vi "KlingerV2 DecodeStatus.vi"(0 "Axe":u8(ring) items=["W", "X", "Y", "Z"], 2 "Message Cont":string caption="Message de statut", 3 "error in":errorcluster) -> (4 "PLimit":bool caption="Limite +", 5 "Moving":bool caption="Déplacement\nen cours", 6 "Position":dbl format="%#.1f", 7 "Statut":bool, 8 "NLimit":bool caption="Limite -", 10 "error out":errorcluster)   [LabVIEW 2012]
doc: "Ce VI décode le message de statut du contrôleur et rapporte les informations pour l'axe désiré"
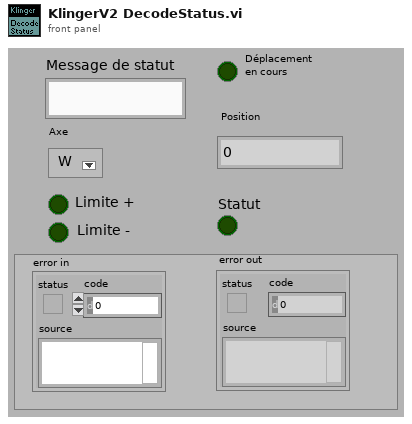
[diagram p1: front panel]
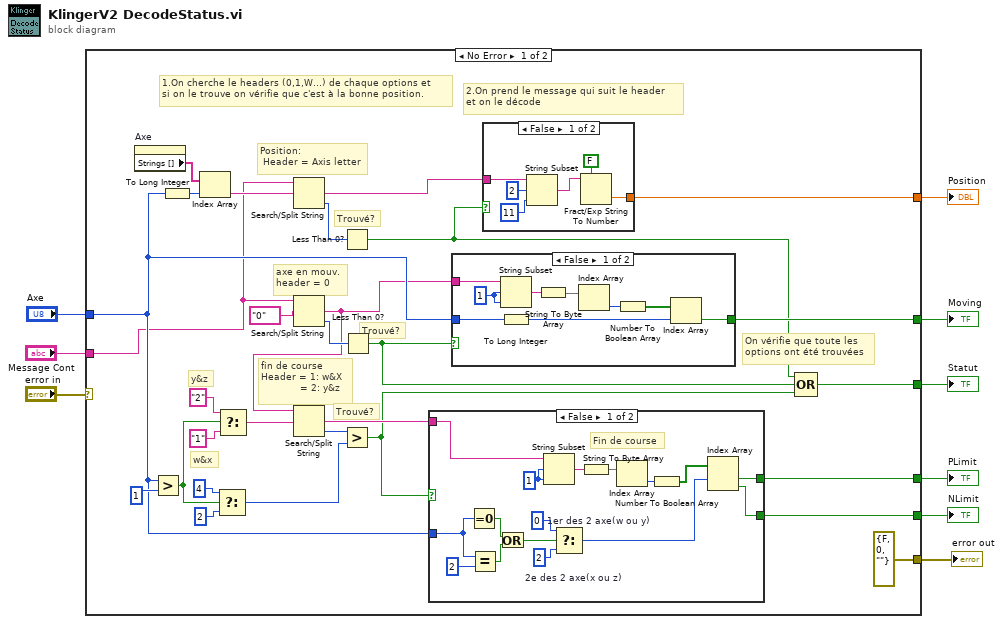
[diagram p0: block diagram]
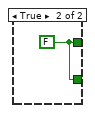
[diagram p2: hidden frame]
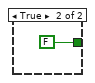
[diagram p3: hidden frame]
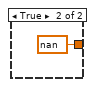
[diagram p4: hidden frame]
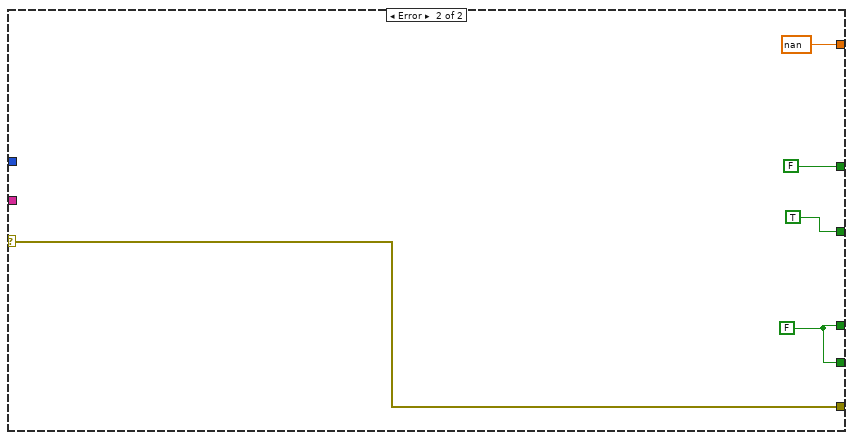
[diagram p5: hidden frame]
diagram:
  n1 = case shown="No Error" "error in" {
    selector: "error in" -> [_ w75]
    tunnel: [w35 nan] -> w9
    tunnel: [w34 FALSE] -> w8
    tunnel: "Axe" -> [w16 _]
    tunnel: [errorcluster {"status"=FALSE, "code"=0, "source"=""} ("error IO") w75] -> w6
    tunnel: [w17 TRUE ("Statut")] -> w5
    tunnel: "Message Cont" -> [w11 _]
    tunnel: [w19 w73] -> w2
    tunnel: [w18 w73] -> w1
    frame No Error {
      # "2.On prend le message qui suit le header \net on le décode"
      # "1.On cherche le headers (0,1,W...) de chaque options et\nsi on le trouve on vérifie que c'est à la bonne position."
      # "Trouvé?"
      # "Trouvé?"
      # "Trouvé?"
      # "On vérifie que toute les \noptions ont été trouvées"
      # "w&x"
      # "y&z"
      # "fin de course\nHeader = 1: w&X\n             = 2: y&z"
      # "Position:\n Header = Axis letter"
      # "axe en mouv.\nheader = 0"
      n2 = property on="Axe" class="Ring (strict)"() -> ("Strings []"=w33:string[])  [unwired: 2 in, 2 out]
      n3 = Greater?(x=w16, y=u8 1) -> (0:w23:bool)
      n4 = To Long Integer(number=w16) -> (32bit integer=w38:i32)
      n5 = Index Array(array=w33, index=w38) -> (element=w37:string)
      n6 = Select(t=4 ("y"), s=w23, f=2 ("y")) -> (s? t:f=w21:i32)
      n7 = Select(t="2" ("search string/char (-)"), s=w23, f="1" ("search string/char (-)")) -> (s? t:f=w22:string)
      n8 = Search/Split String(string=w11, search string/char (-)=w37) -> (match + rest of string=w36:string, offset of match=w32:i32)  [unwired: 1 in, 1 out]
      n9 = Search/Split String(string=w11, search string/char (-)="0") -> (match + rest of string=w10:string, offset of match=w30:i32)  [unwired: 1 in, 1 out]
      n10 = Search/Split String(string=w10, search string/char (-)=w22) -> (match + rest of string=w20:string, offset of match=w29:i32)  [unwired: 1 in, 1 out]
      n11 = Less Than 0?(x=w32) -> (x < 0?=w14:bool)
      n12 = Greater?(x=w29, y=w21) -> (0:w12:bool)
      n13 = Less Than 0?(x=w30) -> (x < 0?=w13:bool)
      n14 = case shown="False" w12 {
        tunnel: w20 -> [w43 _]
        tunnel: [w41 w55] -> w19
        tunnel: [w40 w55] -> w18
        tunnel: w16 -> [w39 _]
        frame False {
          w52 = 2  # 2e des 2 axe(x ou z)
          w53 = 0  # 1er des 2 axe(w ou y)
          w44 = 1 ("offset (0)")
          # "Fin de course"
          n15 = Equal To 0?(x=w39) -> (x = 0?=w51:bool)
          n16 = Equal?(x=w39, y=u8 2) -> (x = y?=w50:bool)
          n17 = Or(x=w51, y=w50) -> (x .or. y?=w48:bool)
          n18 = String Subset(string=w43, offset (0)=w44, length (rest)=w44) -> (substring=w47:string)
          n19 = Select(t=w53, s=w48, f=w52) -> (s? t:f=w42:i32)
          n20 = String To Byte Array(string=w47) -> (unsigned byte array=w46:u8[])
          n21 = Index Array(array=w46) -> (element=w45:u8)  [unwired: 1 in]
          n22 = Number To Boolean Array(number=w45) -> (Boolean array=w54:bool[])
          n23 = Index Array(array=w54, index #1=w42) -> (element #1=w41:bool, element #2=w40:bool)  [unwired: 1 in]
        }
        frame True {
          w55 = FALSE
        }
      }
      n24 = case shown="False" w13 {
        tunnel: [w61 FALSE] -> w34
        tunnel: w10 -> [w59 _]
        tunnel: w16 -> [w56 _]
        frame False {
          w58 = 1 ("offset (0)")
          n25 = String Subset(string=w59, offset (0)=w58, length (rest)=w58) -> (substring=w60:string)
          n26 = To Long Integer(number=w56) -> (32bit integer=w57:i32)
          n27 = String To Byte Array(string=w60) -> (unsigned byte array=w64:u8[])
          n28 = Index Array(array=w64) -> (element=w62:u8)  [unwired: 1 in]
          n29 = Number To Boolean Array(number=w62) -> (Boolean array=w63:bool[])
          n30 = Index Array(array=w63, index=w57) -> (element=w61:bool)
        }
        frame True {
        }
      }
      n31 = case shown="False" w14 {
        tunnel: w36 -> [w68 _]
        tunnel: [w66 nan] -> w35
        frame False {
          n32 = String Subset(string=w68, offset (0)=2, length (rest)=11 ("length (rest)")) -> (substring=w67:string)
          n33 = Fract/Exp String To Number(use system decimal point (T)=FALSE, string=w67) -> (number=w66:dbl)  [unwired: 2 in, 1 out]
        }
        frame True {
        }
      }
      n34 = Compound Arithmetic op=OR(w14, w13, w12) -> (w17:bool)
    }
    frame Error {
      w73 = FALSE
    }
  }
  "Moving" <- w8
  "PLimit" <- w2
  "NLimit" <- w1
  "Position" <- w9
  "error out" <- w6
  "Statut" <- w5
